vi "VT4001_Chamber Open.vi"(8 "error in":errorcluster, 11 "COM VISA Resource":refnum<visa-resource-name>="COM6") -> (0 "error out":errorcluster={"status"=FALSE, "code"=1073676294, "source"="VISA Read in MB Master.lvlib:MB_ADU_RTU.lvclass:RX ADU.vi:4960001->MB Master.lvlib:MB_Master_Serial.lvclass:Querry.vi:3550001->MB Master.lvlib:Write Single Coil.vi:160001->VT4001_Chamber Close.vi"}, 2 "OK":bool=TRUE)   [LabVIEW 2019]
doc: "Modbus Comm Tester\n\nThis VI demonstrates the usage of the Modbus Master API for both TCP and Serial connections.\nIt is also a useful tool for testing communication with your modbus device. You can test different\ncommunication parameters and coil/register address ranges without having to write any code.\n\nCopyright (c) 2016, Plasmionique Inc.\nAll rights reserved.\n\nLicense: BSD (2-Clause) - http://opensource.org/licenses/BSD-2-Clause"
uses:
  <vilib>/Plasmionique/MB Master/MB_Master_Serial/MB_Master_Serial.lvclass
  D:/National Instruments/LabVIEW 2019/vi.lib/Plasmionique/MB Master/MB_Master/MB_Master.lvclass
  <vilib>/Plasmionique/MB Master/MB Master.lvlib
panel:
  # "Communication Settings"
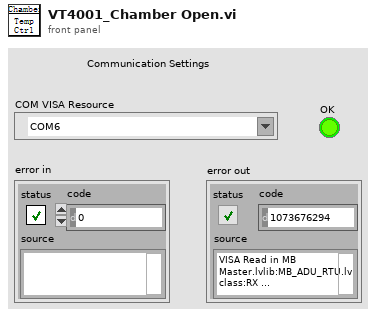
[diagram p1: front panel]
types:
  T1 = cluster{"baud rate (bps)":u32, "stop bits":u16, "parity":u16, "flow control":u16, "timeout":u32, "retries":i32}
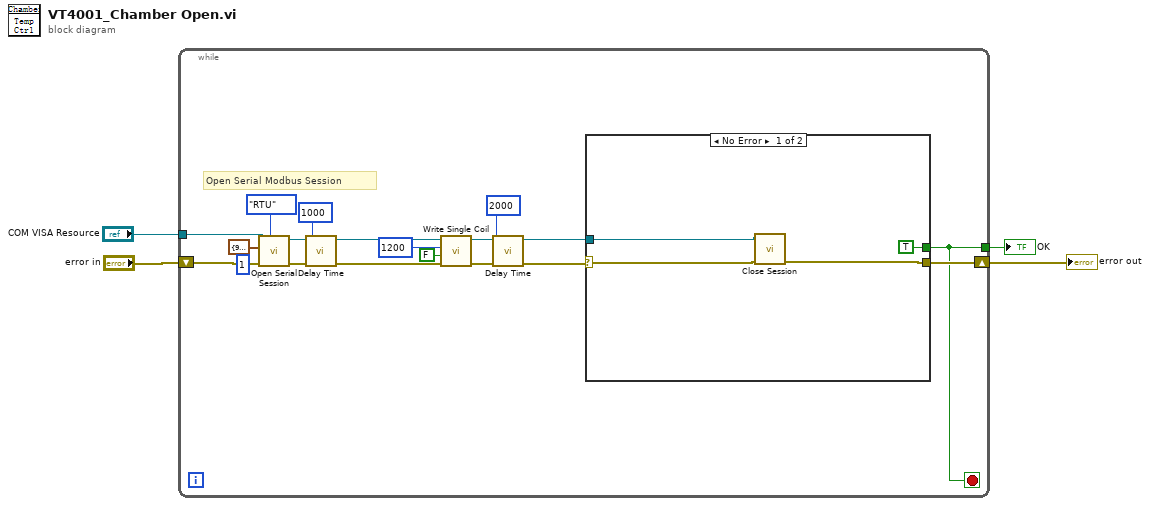
[diagram p0: block diagram]
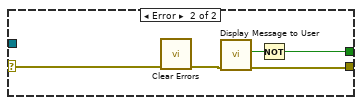
[diagram p2: hidden frame]
diagram:
  n1 = while {
    tunnel: [w5] -> w4
    tunnel: "COM VISA Resource" -> [w18]
    shift-right: [w14] -> w1
    shift-left: "error in" -> [w20]
    stop <- w5 stop-if-true
    # "Open Serial Modbus Session"
    n2 = call <vilib>:"Open Serial Session.vi"("Mode (RTU)"=enum16{"RTU", "ASCII"}."RTU", "Error in"=w20, "Slave ID"=u8 1, "Serial Config"=T1 {"baud rate (bps)"=9600, "stop bits"=10, "parity"=0, "flow control"=0, "timeout"=1000, "retries"=1}, "VISA Resource"=w18) -> ("Error out"=w21:errorcluster, "MB_Serial session"=w8:refnum<class "MB_Master_Serial.lvclass">)  [unwired: 5 in]
    n3 = call "Delay Time.vi"("Error In"=w21, "Delay Time (ms)"=u32 1000) -> ("Error Out"=w9:errorcluster)  [unwired: 9 in]
    n4 = call <vilib>:"Write Single Coil.vi"("error in (no error)"=w9, "value"=FALSE, "address"=u16 1200, "MB session in"=w8) -> ("error out"=w11:errorcluster, "MB session out"=w7:refnum<class "MB_Master_Serial.lvclass">)  [unwired: 6 in]
    n5 = call "Delay Time.vi"("Error In"=w11, "Delay Time (ms)"=u32 2000) -> ("Error Out"=w6:errorcluster)  [unwired: 9 in]
    n6 = case shown="No Error" w6 {
      selector: w6 -> [w25 w27]
      tunnel: w7 -> [w23 _]
      tunnel: [w24 w30] -> w14
      tunnel: [TRUE w28] -> w5
      frame No Error {
        n7 = call-dynamic "Close Session.vi"("error in (no error)"=w25, "MB_Serial session"=w23) -> ("error out"=w24:errorcluster)  [unwired: 9 in]
      }
      frame Error {
        n8 = call <vilib>:"Clear Errors.vi"("error in (no error)"=w27) -> ("error out"=w26:errorcluster)  [unwired: 5 in, 1 out]
        n9 = call "Display Message to User"("error in (no error)"=w26) -> ("error out"=w30:errorcluster, "OK"=w29:bool)  [unwired: 9 in]
        n10 = Not(x=w29) -> (.not. x?=w28:bool)
      }
    }
  }
  "OK" <- w4
  "error out" <- w1
